vi "dribbler.vi"(7 "Parameters.lvclass":refnum<class "Parameters.lvclass">, 8 "error in (no error)":errorcluster, 9 "Ball":refnum<class "Ball.lvclass">, 10 "Robot":refnum<class "Robot.lvclass">, 11 "Utilities in":refnum<class "Utilities.lvclass">) -> (0 "error out":errorcluster, 2 "Dribbler?":bool, 3 "Utilities out":refnum<class "Utilities.lvclass">)   [LabVIEW 2020, in "Utilities.lvclass"]
uses:
  Utilities.lvclass
  Robot_class/Robot.lvclass
  C:/Users/anton/Desktop/RoboIME/IC/SSL_AI/Object_class/Object.lvclass
  Ball_class/Ball.lvclass
  Parameters_class/Parameters.lvclass
  Parameters_class/Parameters.lvclass/Parameters.ctl
  Object_class/Object.lvclass/Object.ctl
  Object_class/Read x.vi
  Object_class/Read y.vi
  Parameters_class/Read Dribbler.vi
  Parameters_class/Read distToActivateDibbler.vi
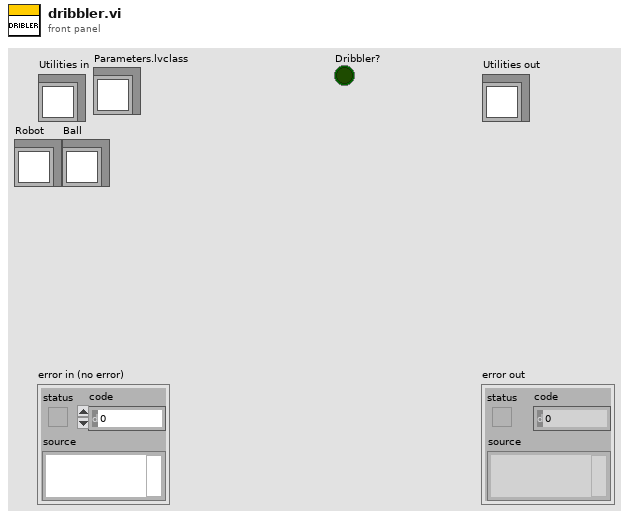
[diagram p1: front panel]
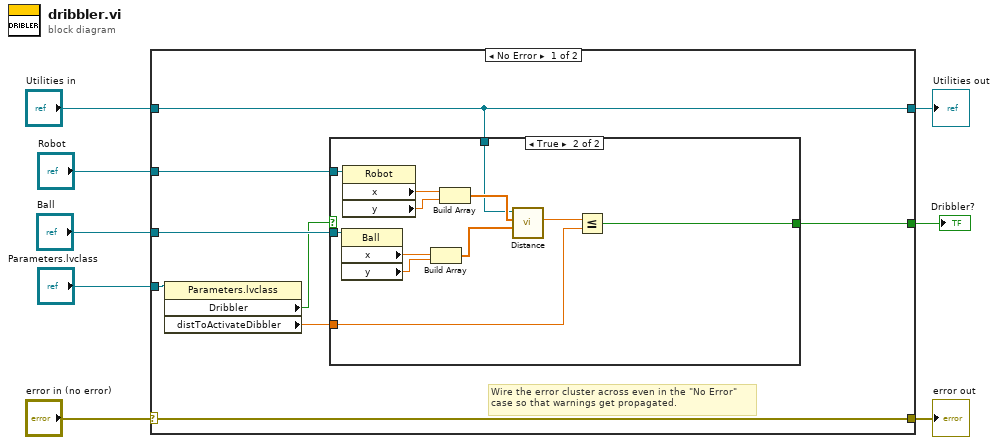
[diagram p0: block diagram]
diagram:
  n1 = case shown="No Error" "error in (no error)" {
    selector: "error in (no error)" -> [w16 w31]
    tunnel: [w16 w31] -> w7
    tunnel: [w13 w30] -> w5
    tunnel: "Utilities in" -> [w13 w30]
    tunnel: "Robot" -> [w15 _]
    tunnel: "Ball" -> [w14 _]
    tunnel: [w12 _] -> w2
    tunnel: "Parameters.lvclass" -> [w11 _]
    frame No Error {
      # "Wire the error cluster across even in the \"No Error\"\ncase so that warnings get propagated."
      n2 = property class="Parameters.lvclass"(reference=w11) -> ("Dribbler"=w10:bool, "distToActivateDibbler"=w9:dbl)  [unwired: 1 in, 2 out]
      n3 = case shown="True" w10 {
        selector: w10 -> [w17 _]
        tunnel: w15 -> [_ w29]
        tunnel: w14 -> [_ w28]
        tunnel: w13 -> [_ w21]
        tunnel: [w17 w19] -> w12
        tunnel: w9 -> [_ w18]
        frame False {
        }
        frame True {
          n4 = property class="Ball"(reference=w28) -> ("x"=w25:dbl, "y"=w24:dbl)  [unwired: 1 in, 2 out]
          n5 = property class="Robot"(reference=w29) -> ("x"=w27:dbl, "y"=w26:dbl)  [unwired: 1 in, 2 out]
          n6 = Build Array(w25, w24) -> (w22:dbl[])
          n7 = Build Array(w27, w26) -> (w23:dbl[])
          n8 = call "Distance.vi"("P1"=w22, "P2"=w23, "Utilities in"=w21) -> ("Distance"=w20:dbl)  [unwired: 6 in, 2 out]
          n9 = Less Or Equal?(x=w20, y=w18) -> (x <= y?=w19:bool)
        }
      }
    }
    frame Error {
    }
  }
  "error out" <- w7
  "Utilities out" <- w5
  "Dribbler?" <- w2
